vi "Start Buzzer Acquisition.vi"(8 "error in (no error)":errorcluster, 10 "Simulated?":bool, 11 "Controller in":refnum<class "Controller.lvclass">) -> (0 "error out":errorcluster, 3 "Controller out":refnum<class "Controller.lvclass">)   [LabVIEW 2024, in "Controller.lvlib" / "Controller.lvclass"]
uses:
  Controller.lvclass
  C:/Program Files/National Instruments/LabVIEW 2024/vi.lib/ActorFramework/Actor/Actor.lvclass
  Simulated HW/Simulated Hardware/Simulated Hardware.lvclass
  Hardware Buzzer/Hardware Buzzer/Hardware Buzzer.lvclass
  Controller.lvclass/Controller.ctl
  Hardware Buzzer/Hardware Buzzer/Hardware Buzzer.lvclass/Hardware Buzzer.ctl
  <vilib>/ActorFramework/Message Enqueuer/Message Enqueuer.lvclass/Message Enqueuer.ctl
  <vilib>/ActorFramework/Message Enqueuer/Enqueue.vi
  <vilib>/ActorFramework/Stop Msg/Stop Msg.lvclass
  C:/Program Files/National Instruments/LabVIEW 2024/vi.lib/ActorFramework/Message/Message.lvclass
  <vilib>/ActorFramework/Message Priority Queue/Priority Enqueue.vi
  <vilib>/ActorFramework/Actor/Actor.lvclass
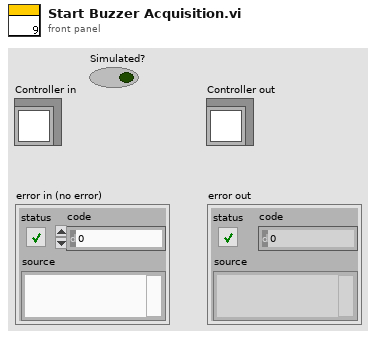
[diagram p1: front panel]
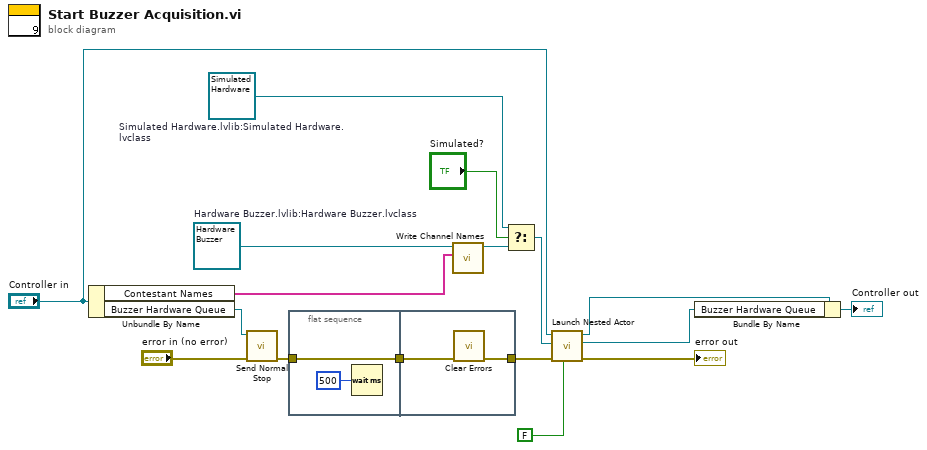
[diagram p0: block diagram]
diagram:
  w5 = refnum<class "Hardware Buzzer.lvclass"> refnum  # Hardware Buzzer.lvlib:Hardware Buzzer.lvclass
  w7 = refnum<class "Simulated Hardware.lvclass"> refnum  # Simulated Hardware.lvlib:Simulated Hardware.lvclass
  n1 = Unbundle By Name("Controller in") -> ("Contestant Names"=w3:string[], "Buzzer Hardware Queue"=w11:refnum<class "Message Enqueuer.lvclass">)
  n2 = call <vilib>:"Send Normal Stop.vi"("error in (no error)"="error in (no error)", "Message Enqueuer"=w11) -> ("error out"=w2:errorcluster)  [unwired: 9 in]
  n3 = flat-sequence {
    tunnel: w2 -> [w19]
    tunnel: [w19] -> w1
    tunnel: [w21] -> w10
    tunnel: w1 -> [w20]
    frame #0 {
      n4 = Wait (ms)(milliseconds to wait=u32 500) -> ()  [unwired: 1 out]
    }
    frame #1 {
      n5 = call <vilib>:"Clear Errors.vi"("error in (no error)"=w20) -> ("error out"=w21:errorcluster)  [unwired: 5 in, 1 out]
    }
  }
  n6 = call "Write Channel Names.vi"("Channel Names"=w3, "Hardware Buzzer in"=w5) -> ("Hardware Buzzer out"=w4:refnum<class "Hardware Buzzer.lvclass">)  [unwired: 8 in, 1 out]
  n7 = Select(t=w7, s="Simulated?", f=w4) -> (s? t:f=w6:refnum<class "Actor.lvclass">)
  n8 = call <vilib>:"Launch Nested Actor.vi"("Open Actor Core front panel? (F)"=FALSE, "error in (no error)"=w10, "Nested Actor"=w6, "Caller Actor in"="Controller in") -> ("error out"=→"error out":errorcluster, "Nested Actor's Enqueuer"=w17:refnum<class "Message Enqueuer.lvclass">, "Caller Actor out"=w15:refnum<class "Controller.lvclass">)  [unwired: 5 in]
  n9 = Bundle By Name(cluster=w15, "Buzzer Hardware Queue"=w17) -> (→"Controller out":refnum<class "Controller.lvclass">)
